vi "Add Row.vi"(8 "error in":errorcluster, 10 "RowIndex":i32, 11 "Worksheet in":refnum<k24>) -> (0 "error out":errorcluster, 2 "Row":refnum<k24>, 3 "Worksheet out":refnum<k24>)   [LabVIEW 2019, in "Open Xml.lvlib"]
uses:
  Open Xml.lvlib
  D:/git/Open-Xml-LabVIEW/Source/DocumentFormat.OpenXml.dll
  DocumentFormat.OpenXml.dll
  D:/git/Open-Xml-LabVIEW/Source/OpenXmlGenericsWrapper.dll
  OpenXmlGenericsWrapper.dll
  D:/git/Open-Xml-LabVIEW/Source/DocumentFormat.OpenXml.Framework.dll
  DocumentFormat.OpenXml.Framework.dll
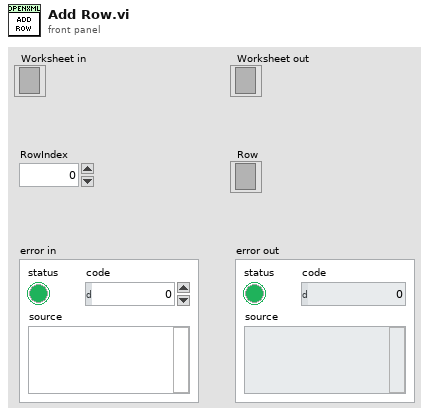
[diagram p1: front panel]
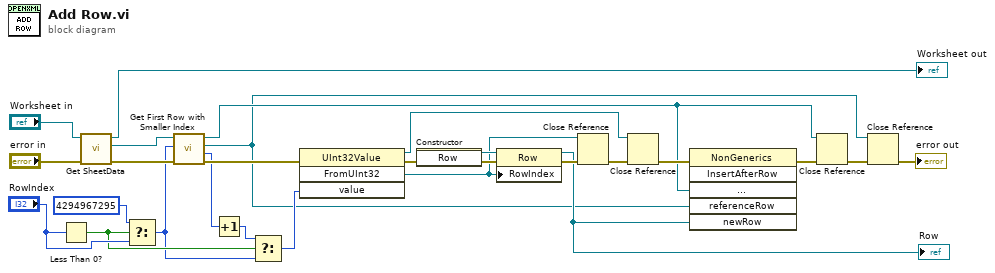
[diagram p0: block diagram]
diagram:
  n1 = Less Than 0?(x="RowIndex") -> (x < 0?=w8:bool)
  n2 = call "Get SheetData.vi"("error in"="error in", "Worksheet in"="Worksheet in") -> ("error out"=w13:errorcluster, "SheetData"=w15:refnum<k24>, "Worksheet out"=→"Worksheet out":refnum<k24>)  [unwired: 7 in]
  n3 = Select(t=u32 4294967295 ("Row Index"), s=w8, f="RowIndex") -> (s? t:f=w6:u32)
  n4 = call "Get First Row with Smaller Index.vi"("error in"=w13, "Row Index"=w6, "SheetData in"=w15) -> ("error out"=w12:errorcluster, "Smaller Row Index"=w9:u32, "Row"=w1:refnum<k24>, "SheetData out"=w2:refnum<k24>)  [unwired: 5 in]
  n5 = Increment(x=w9) -> (x+1=w7:u32)
  n6 = Select(t=w7, s=w8, f=w6) -> (s? t:f=w5:u32)
  n7 = invoke class="UInt32Value" method="FromUInt32"(error in=w12, "value"=w5) -> (reference out=w22:refnum<k24>, error out=w21:errorcluster, "FromUInt32"=w17:refnum<k24>)  [unwired: 2 in, 1 out]
  n8 = constructor class="Row"(error in=w21) -> (reference out=w24:refnum<k24>, error out=w20:errorcluster)  [unwired: 2 in, 1 out]
  n9 = property class="Row"(reference=w24, error in=w20, "RowIndex"=w17) -> (reference out=w3:refnum<k24>, error out=w23:errorcluster)
  "Row" <- w3
  n10 = Close Reference(reference=w17, error in (no error)=w23) -> (error out=w18:errorcluster)
  n11 = Close Reference(reference=w22, error in (no error)=w18) -> (error out=w4:errorcluster)
  n12 = invoke class="NonGenerics" method="InsertAfterRow"(error in=w4, "sheetData"=w2, "referenceRow"=w1, "newRow"=w3) -> (error out=w27:errorcluster)  [unwired: 2 in, 5 out]
  n13 = Close Reference(reference=w2, error in (no error)=w27) -> (error out=w19:errorcluster)
  n14 = Close Reference(reference=w1, error in (no error)=w19) -> (error out=→"error out":errorcluster)
